vi "apFFT.vi"(8 "error in":errorcluster, 9 "1-D Array of Real 2":dbl[](array[numeric]), 11 "string":string="XBR8161") -> (0 "error out":errorcluster, 1 "1-D Array of Real":dbl[](array[numeric]), 3 "string 2":string="XBR8161")   [LabVIEW 2020]
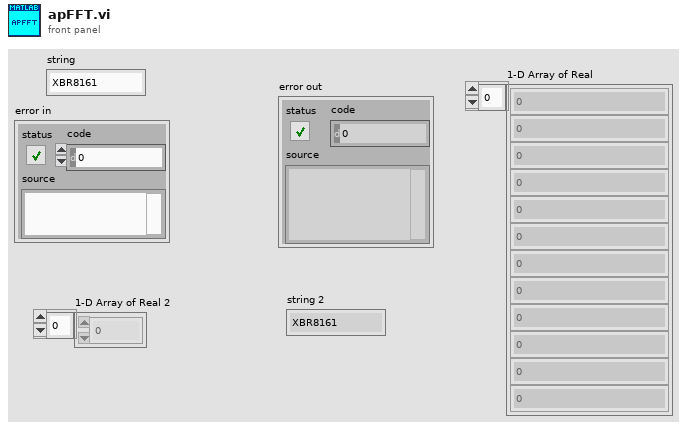
[diagram p1: front panel]
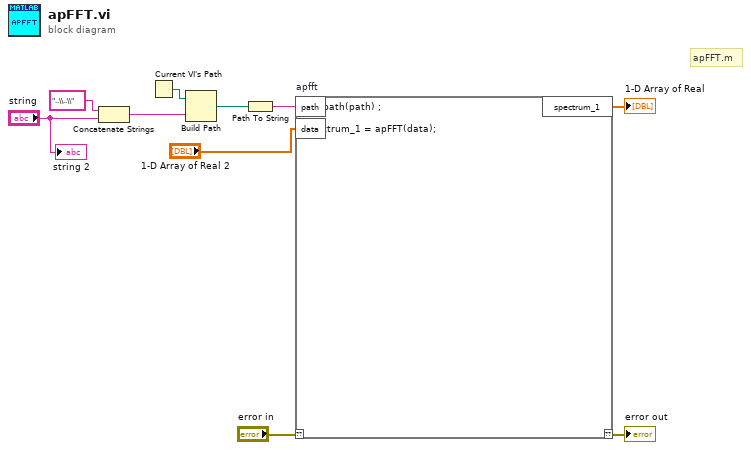
[diagram p0: block diagram]
diagram:
  # "apFFT.m"
  n1 = Concatenate Strings("..\\..\\" ("string"), "string") -> (w1:string)
  n2 = Current VI's Path() -> (path=w8:path)
  n3 = Build Path(base path=w8, name or relative path=w1) -> (appended path=w7:path)
  n4 = Path To String(path=w7) -> (string=w9:string)
  n5 = script code="addpath(path) ;\n\nspectrum_1 = apFFT(data);" "apfft"("??"="error in", "data"="1-D Array of Real 2", "path"=w9) -> ("??"=→"error out":errorcluster, "spectrum_1"=→"1-D Array of Real":dbl[])
  "string 2" <- "string"
